vi "mech366lab1.vi"() -> ()   [LabVIEW 2018]
panel:
  in  "stop":bool
  out "Tank Level Display":cluster{dbl, dbl}(graph)
  out "Tank B":dbl(slide) scale=0.0..25.0
  out "Tank A":dbl(slide) scale=0.0..25.0
  out "Time (s)":dbl
  out "Volts B":dbl
  out "Volts A":dbl
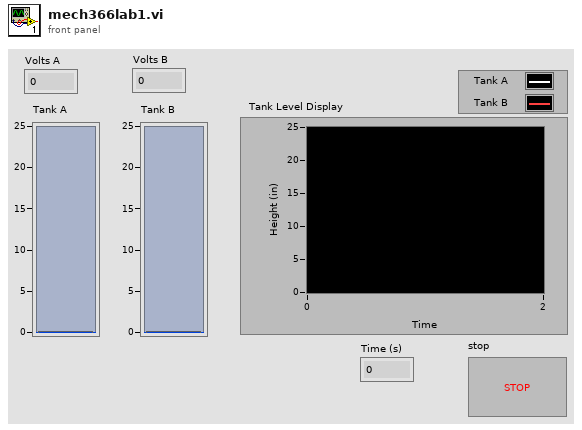
[diagram p1: front panel]
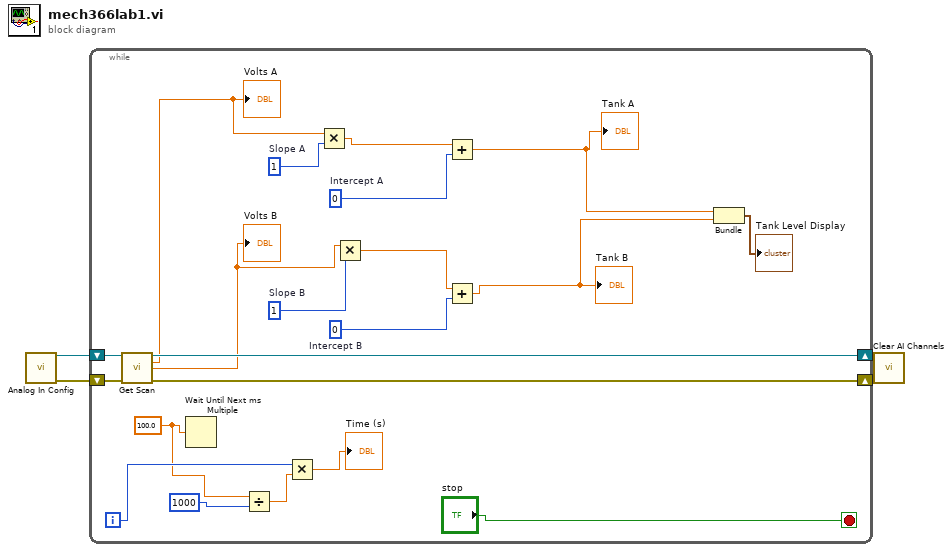
[diagram p0: block diagram]
diagram:
  n1 = call "Analog In Config.vi"() -> ("Refnum out"=w4:refnum<k21>, "error out"=w2:errorcluster)  [unwired: 14 in]
  n2 = while {
    shift-right: [w24] -> w3
    shift-left: w4 -> [w25]
    shift-right: [w22] -> w1
    shift-left: w2 -> [w23]
    i -> [w8]
    stop <- "stop" stop-if-true
    w7 = 100.0
    w18 = 0  # Intercept A
    w13 = 0  # Intercept B
    w15 = 1  # Slope B
    w20 = 1  # Slope A
    n3 = call "Get Scan.vi"("Refnum in"=w25, "error in (no error)"=w23) -> ("Refnum out"=w24:refnum<k21>, "Channel A"=w21:dbl, "Channel B"=w16:dbl, "error out"=w22:errorcluster)  [unwired: 10 in]
    "Volts A" <- w21
    "Volts B" <- w16
    n4 = Wait Until Next ms Multiple(millisecond multiple=w7) -> ()  [unwired: 1 out]
    n5 = Divide(x=w7, y=1000) -> (x/y=w9:dbl)
    n6 = Multiply(x=w8, y=w9) -> (x*y=→"Time (s)":dbl)
    n7 = Multiply(x=w21, y=w20) -> (x*y=w19:dbl)
    n8 = Multiply(x=w16, y=w15) -> (x*y=w14:dbl)
    n9 = Add(x=w19, y=w18) -> (x+y=w17:dbl)
    "Tank A" <- w17
    n10 = Add(x=w14, y=w13) -> (x+y=w12:dbl)
    "Tank B" <- w12
    n11 = Bundle(w17, w12) -> (→"Tank Level Display":cluster{dbl, dbl})  [unwired: 1 in]
  }
  n12 = call "Clear AI Channels.vi"("Refnum in"=w3, "error in (no error)"=w1) -> ()  [unwired: 14 in]
